vi "Logging Open.vi"(6 "Mode":enum16{"Create", "Open"}(ring), 7 "error in (no error)":errorcluster, 8 "Number":i32, 9 "name":string="log", 10 "base path":path=path "c:/logs") -> (0 "error out":errorcluster, 3 "LoggingDevRef":T1)   [LabVIEW 2012, in "femtoRoboLib.lvlib"]
doc: "Open a Logging reference. \n\nIf <b>Mode</b> is Create, will create a new log at <b>base path</b> named \"<<b>name</b>>.<smallest unused number starting at <b>Number</b>>.log\". e.g. blah.005.log\n\nIf <b>Mode</b> is Open, then it simply opens the log at <b>base path</b> with the literal name <b>name</b>\n\nThe default <b>name</b> is \"log\", and the default <b>base path</b> is \"c:\\logs\". If <b>base path</b> does not exist, it will attempt to create it."
uses:
  femtoRoboLib.lvlib
  Controls/LoggingDevRef.ctl
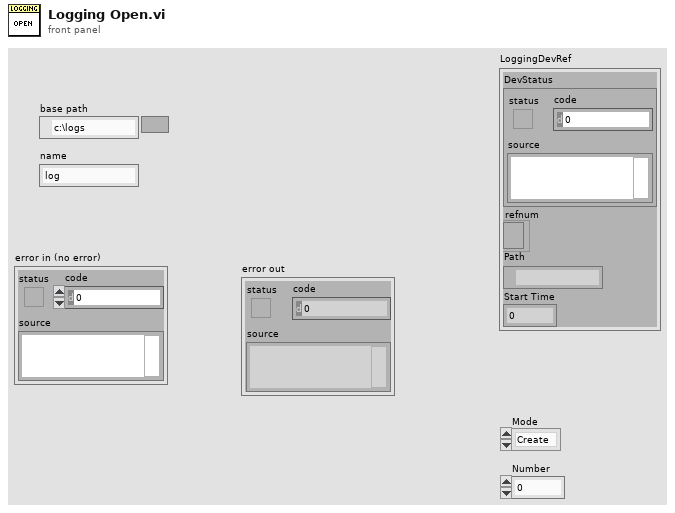
[diagram p1: front panel]
types:
  T1 = typedef "femtoRoboLib.lvlib/LoggingDevRef.ctl" = cluster{"DevStatus":errorcluster, "refnum":refnum<file>, "Path":path, "Start Time":u32}
  T2 = enum16{"open", "replace", "create", "open or create", "replace or create", "replace or create with confirmation"}
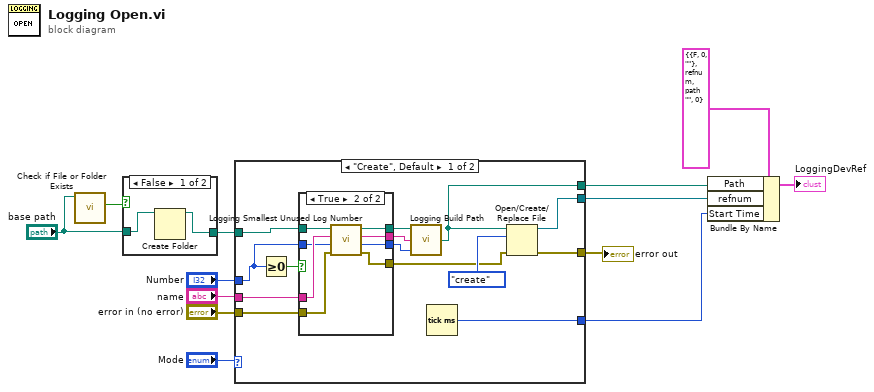
[diagram p0: block diagram]
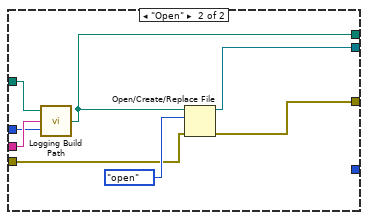
[diagram p4: hidden frame]
diagram:
  n1 = call <vilib>:"Check if File or Folder Exists.vi"("path"="base path") -> ("file or folder exists?"=w12:bool)  [unwired: 8 in, 2 out]
  n2 = case shown="False" w12 {
    tunnel: "base path" -> [w15 w16]
    tunnel: [w14 w16] -> w11
    frame False {
      n3 = Create Folder(path (use dialog)=w15) -> (created path=w14:path)  [unwired: 2 in, 2 out]
    }
    frame True {
    }
  }
  n4 = case shown="\"Create\", Default" "Mode" {
    tunnel: [w30 w50] -> w6
    tunnel: w11 -> [w26 w48]
    tunnel: "name" -> [w25 w47]
    tunnel: [w20 w43] -> w7
    tunnel: [w28 _] -> w5
    tunnel: "Number" -> [w22 w46]
    tunnel: "error in (no error)" -> [w24 w45]
    tunnel: [w18 w44] -> w1
    frame "Create", Default {
      n5 = Greater Or Equal To 0?(x=w22) -> (x >= 0?=w27:bool)
      n6 = case shown="True" w27 {
        tunnel: w26 -> [w33 w41]
        tunnel: w25 -> [w31 w40]
        tunnel: w24 -> [w32 w42]
        tunnel: [w33 w36] -> w23
        tunnel: w22 -> [w34 w39]
        tunnel: [w34 w37] -> w21
        tunnel: [w32 w38] -> w19
        tunnel: [w31 w35] -> w17
        frame False {
        }
        frame True {
          n7 = call "Logging Smallest Unused Log Number.vi"("error in (no error)"=w42, "Starting Offset"=w39, "name"=w40, "base path"=w41) -> ("error out"=w38:errorcluster, "Number"=w37:i32, "name out"=w35:string, "base path out"=w36:path)  [unwired: 4 in]
        }
      }
      n8 = call "Logging Build Path.vi"("number"=w21, "name"=w17, "base path"=w23) -> ("built path"=w20:path)
      n9 = Tick Count (ms)() -> (millisecond timer value=w28:u32)
      n10 = Open/Create/Replace File(file path (use dialog)=w20, error in=w19, operation (0:open)=T2."create") -> (refnum out=w30:refnum<file>, error out=w18:errorcluster)  [unwired: 3 in, 1 out]
    }
    frame "Open" {
      n11 = call "Logging Build Path.vi"("number"=w46, "name"=w47, "base path"=w48) -> ("built path"=w43:path)
      n12 = Open/Create/Replace File(file path (use dialog)=w43, error in=w45, operation (0:open)=T2."open") -> (refnum out=w50:refnum<file>, error out=w44:errorcluster)  [unwired: 3 in, 1 out]
    }
  }
  "error out" <- w1
  n13 = Bundle By Name(cluster=T1 {"DevStatus"={"status"=FALSE, "code"=0, "source"=""}, "refnum"=refnum, "Path"=path "", "Start Time"=0} ("LoggingDevRef"), "Path"=w7, "refnum"=w6, "Start Time"=w5) -> (→"LoggingDevRef":T1)
